vi "multiplier to color converter.vi"(2 "Multiplier select":T1) -> (6 "Multiplier color":u32(colorbox))   [LabVIEW 2018]
uses:
  multiplier--control.ctl
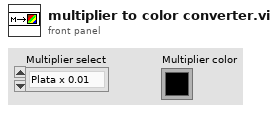
[diagram p1: front panel]
types:
  T1 = typedef "multiplier--control.ctl" = enum16{"Plata x 0.01", "Oro x 0.1 ", "Negro - x 1", "Marrón - x 10", "Rojo - x 100", "Naranja - x 1k", "Amarillo - x 10k", "Verde - 100k", "Azul - x 1M", "Violeta - x10 M", "Gris - x 100M", "Blanco - x 1G"}
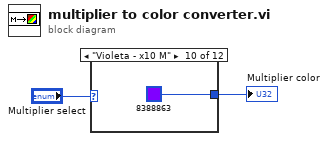
[diagram p0: block diagram]
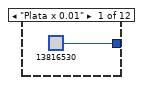
[diagram p2: hidden frame]
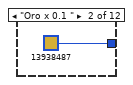
[diagram p3: hidden frame]
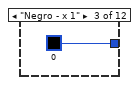
[diagram p4: hidden frame]
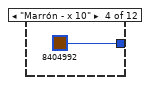
[diagram p5: hidden frame]
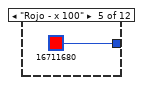
[diagram p6: hidden frame]
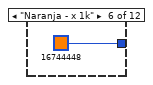
[diagram p7: hidden frame]
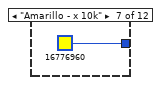
[diagram p8: hidden frame]
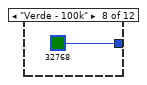
[diagram p9: hidden frame]
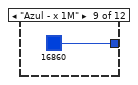
[diagram p10: hidden frame]
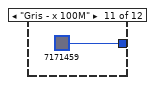
[diagram p11: hidden frame]
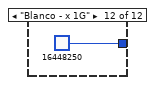
[diagram p12: hidden frame]
diagram:
  n1 = case shown="\"Violeta - x10 M\"" "Multiplier select" {
    tunnel: [u32 13816530 u32 13938487 u32 0 u32 8404992 u32 16711680 u32 16744448 u32 16776960 u32 32768 u32 16860 u32 8388863 u32 7171459 u32 16448250] -> w1
    frame "Plata x 0.01" {
    }
    frame "Oro x 0.1 " {
    }
    frame "Negro - x 1" {
    }
    frame "Marrón - x 10" {
    }
    frame "Rojo - x 100" {
    }
    frame "Naranja - x 1k" {
    }
    frame "Amarillo - x 10k" {
    }
    frame "Verde - 100k" {
    }
    frame "Azul - x 1M" {
    }
    frame "Violeta - x10 M" {
    }
    frame "Gris - x 100M" {
    }
    frame "Blanco - x 1G" {
    }
  }
  "Multiplier color" <- w1
